vi "WriteDestinations.vi"(8 "Error In":errorcluster, 10 "Destinations":string[](array[string]), 11 "object in":refnum<class "Module.lvclass">) -> (0 "Error Out":errorcluster, 3 "object out":refnum<class "Module.lvclass">)   [LabVIEW 2021, in "Module.lvclass"]
uses:
  Module.lvclass
  Module.lvclass/Module.ctl
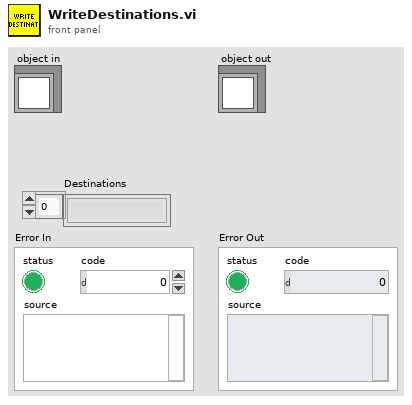
[diagram p1: front panel]
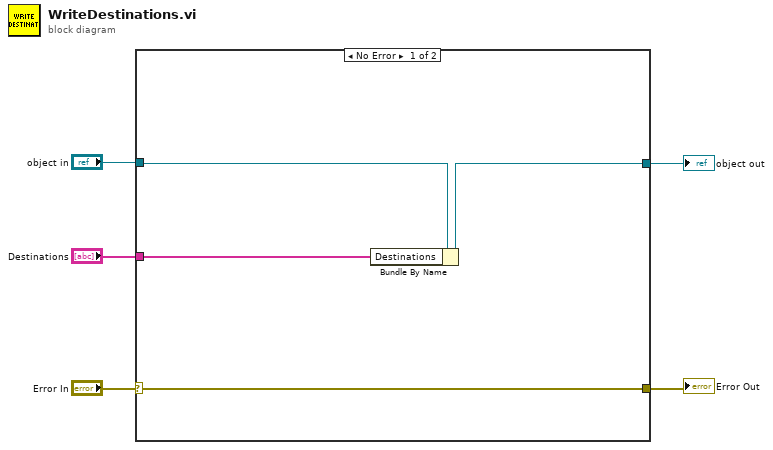
[diagram p0: block diagram]
diagram:
  n1 = case shown="No Error" "Error In" {
    selector: "Error In" -> [w8 w11]
    tunnel: [w8 w11] -> w4
    tunnel: [w6 w10] -> w2
    tunnel: "object in" -> [w7 w10]
    tunnel: "Destinations" -> [w9 _]
    frame No Error {
      n2 = Bundle By Name(cluster=w7, "Destinations"=w9) -> (w6:refnum<class "Module.lvclass">)
    }
    frame Error {
    }
  }
  "Error Out" <- w4
  "object out" <- w2
